vi "INSERT_SENSOR.vi"(8 "error in (no error)":errorcluster, 10 "Sensor Data in":T1, 11 "Refnum in":T2) -> (0 "error out":errorcluster, 2 "Sensor Data out":T1, 3 "Refnum out":T2)   [LabVIEW 2018, in "MySQLTools.lvlib"]
uses:
  MySQLTools.lvlib
  TypeDefs/Sensor Data.ctl
  <vilib>/addons/database/Connection.llb/Conn ObjectReference.ctl
  <vilib>/addons/database/NI_Database_API.lvlib
panel:
  in  "Stop":bool
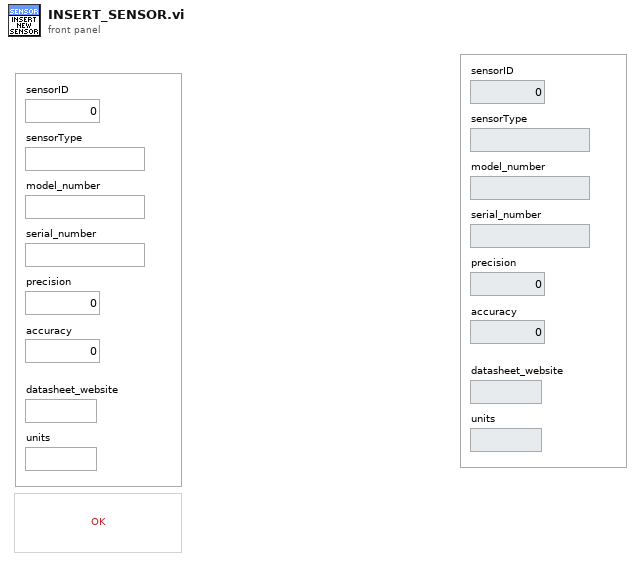
[diagram p1: front panel]
types:
  T1 = typedef "MySQLTools.lvlib/Sensor Data.ctl" = cluster{"sensorID":u16, "sensorType":string, "model_number":string, "serial_number":string, "precision":dbl, "accuracy":dbl, "datasheet_website":string, "units":string}
  T2 = typedef "NI_Database_API.lvlib/Conn ObjectReference.ctl" = refnum<k1>
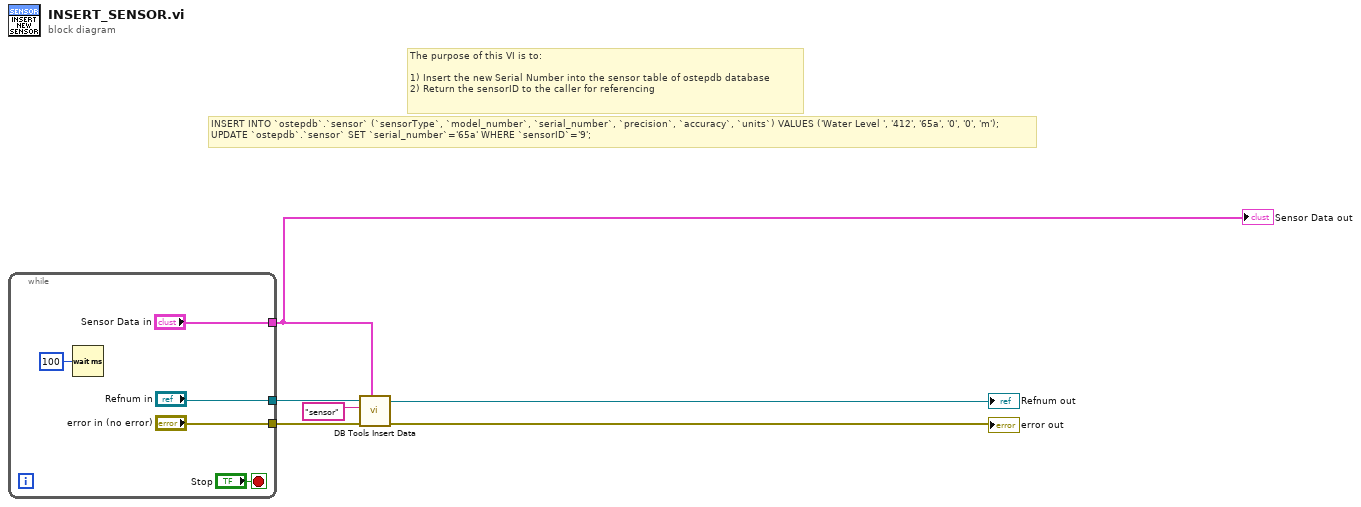
[diagram p0: block diagram]
diagram:
  # "INSERT INTO `ostepdb`.`sensor` (`sensorType`, `model_number`, `serial_number`, `precision`, `accuracy`, `units`) VALUES ('Water Level ', '412', '65a', '0', '0', 'm');\nUPDATE `ostepdb`.`sensor` SET `serial_number`='65a' WHERE `sensorID`='9';"
  # "The purpose of this VI is to:\n\n1) Insert the new Serial Number into the sensor table of ostepdb database\n2) Return the sensorID to the caller for referencing"
  n1 = while {
    tunnel: ["Refnum in"] -> w4
    tunnel: ["error in (no error)"] -> w3
    tunnel: ["Sensor Data in"] -> w2
    stop <- "Stop" stop-if-true
    n2 = Wait (ms)(milliseconds to wait=u32 100) -> ()  [unwired: 1 out]
  }
  "Sensor Data out" <- w2
  n3 = call <vilib>:"DB Tools Insert Data.vi"("data"=w2, "error in (no error)"=w3, "table"="sensor", "connection reference"=w4) -> ("error out"=→"error out":errorcluster, "connection reference out"=→"Refnum out":T2)  [unwired: 6 in]
